vi "CliReadSZLList.vi"(0 "ref in":u64, 11 "error in (no error)":errorcluster) -> (4 "ref out":u64, 6 "Result":i32, 13 "ItemsCount":i32, 14 "List":u16[](array[numeric]), 15 "error out":errorcluster)   [LabVIEW 2016, in "Snap7.lvlib"]
uses:
  Snap7.lvlib
  win32/lv_snap7.dll
panel:
  in  "var Size":i32
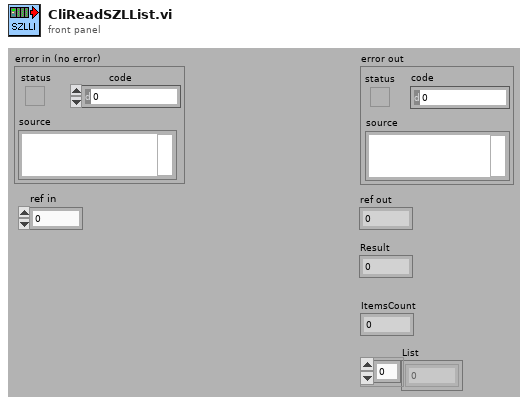
[diagram p1: front panel]
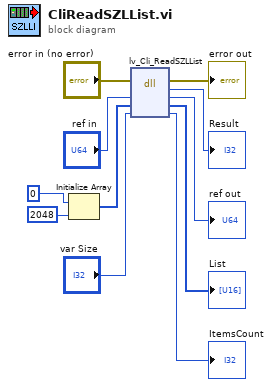
[diagram p0: block diagram]
diagram:
  n1 = Initialize Array(u16 0, 2048) -> (w4:u16[])
  n2 = dll-call lib="D:/maszup/svn/LineTraceSystem/SOFTWARE/sources/Drivers/PLC/Snap7/lib/win32/lv_snap7.dll" fn="lv_Cli_ReadSZLList"(error in="error in (no error)", "Client"="ref in", "pUsrData"=w4, "ItemsCount"="var Size") -> (error out=→"error out":errorcluster, "return type"=→"Result":i32, "Client"=→"ref out":u64, "pUsrData"=→"List":u16[], "ItemsCount"=→"ItemsCount":i32)  [unwired: 2 in, 1 out]
